vi "Read Data Bits.vi"(8 "error in (no error)":errorcluster, 11 "RTU data unit in":refnum<class "RTU Data Unit.lvclass">) -> (0 "error out":errorcluster, 2 "data bits":u16=8, 3 "RTU data unit out":refnum<class "RTU Data Unit.lvclass">)   [LabVIEW 2020, in "SubVIs.lvlib" / "RTU Data Unit.lvclass"]
doc: "Acts as a constant, and provides a way for the serial slave to properly configure the serial interface. 8 bits in this case."
uses:
  <vilib>/Modbus/subvis/Transmission Data Unit (ADU)/RTU Data Unit/RTU Data Unit.lvclass
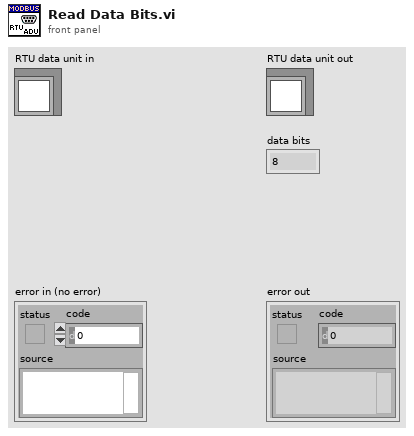
[diagram p1: front panel]
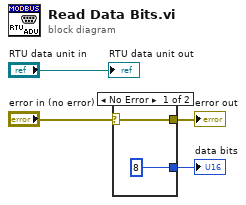
[diagram p0: block diagram]
diagram:
  n1 = case shown="No Error" "error in (no error)" {
    selector: "error in (no error)" -> [w5 w7]
    tunnel: [u16 8 ("data bits") _] -> w3
    tunnel: [w5 w7] -> w1
    frame No Error {
    }
    frame Error {
    }
  }
  "error out" <- w1
  "data bits" <- w3
  "RTU data unit out" <- "RTU data unit in"
